vi "Drive Train.vi"(11 "Refnum in":refnum<k33>) -> ()   [LabVIEW 2014]
uses:
  TeleopCmd.ctl
  CmdFlag.ctl
  Drive Train Metrics.ctl
  <vilib>/Platform/TimedLoop/XDataNode/timing_clust.ctl
  <vilib>/Platform/TimedLoop/XDataNode/nitl_modes.ctl
  <vilib>/Platform/TimedLoop/XDataNode/wakeup.ctl
  <vilib>/platform/TimedLoop/XDataNode/XDataNode.xnode
  <vilib>/Platform/TimedLoop/XDataNode/XDNodeRunTimeDep.lvlib
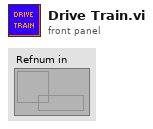
[diagram p1: front panel]
types:
  T1 = typedef "Drive Train Metrics.ctl" = cluster{"CmdFlag":T2, "Right Motor Power":dbl, "Left Motor Power":dbl, "Filtered Left Drive Rate":dbl, "Filtered Right Drive Rate":dbl, "Time of Last Metric":u32, "FIFO Timeout":i32, "Requested Left Velocity":dbl, "Requested Right Velocity":dbl, "throttle":dbl, "turn":dbl, "MaxDrivePwr":dbl, "Strafe":dbl, "Override":bool, "Time Of Last Turn":dbl, "Front_Strafe_Power":dbl, "Back_Strafe_Power":dbl, "MaxStrafePwr":dbl, "PrevMotorLevel":u8}
  T2 = typedef "CmdFlag.ctl" = enum16{"noop", "logflag", "suspend", "resume"}
  T3 = typedef "XDNodeRunTimeDep.lvlib/timing_clust.ctl" = cluster{"Expected End [f-1]":u64, "Actual End [f-1]":u64, "Finished Late? [f-1]":bool, "Expected End [i-1]":u64, "Actual End [i-1]":u64, "Finished Late? [i-1]":bool, "Expected Start [i]":u64, "Actual Start [i]":u64, "Expected Start [f]":u64, "Actual Start [f]":u64, "Source Name":string, "Structure Name":string, "Period":i64, "Deadline":i64, "Offset":i64, "Start":i64, "Priority":i32, "Timeout":i32, "Mode":T4, "Wakeup Reason":T5, "Error":errorcluster, "Source Type":string, "Secondary Source Type":string, "Global End Time":u64, "Global Start Time":u64, "Frame Duration":u64, "Iteration Duration":u64, "Assigned CPU":i32, "I/O Scan Engine Mode":u32}
  T4 = typedef "XDNodeRunTimeDep.lvlib/nitl_modes.ctl" = enum32{"No Change", "Process missed periods, maintain original phase", "Discard missed periods, maintain original phase", "Process missed periods, ignore original phase", "Discard missed periods, ignore original phase"}
  T5 = typedef "XDNodeRunTimeDep.lvlib/wakeup.ctl" = enum32{"Normal", "Aborted", "Asynchronous wakeup", "Timing source error", "Timed loop error", "Timeout"}
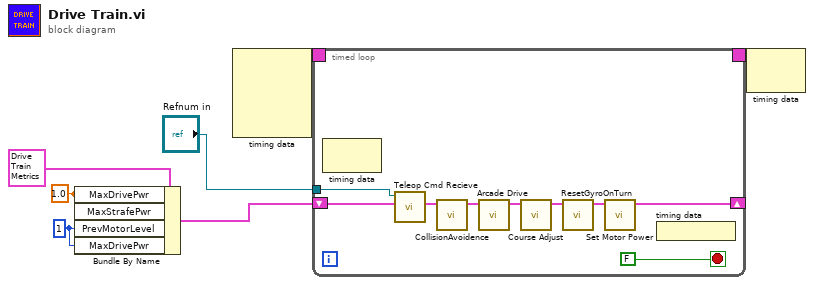
[diagram p0: block diagram]
diagram:
  w1 = u8 1 ("PrevMotorLevel")
  w2 = 1.0 ("MaxMotorPwr")
  n1 = Bundle By Name(cluster=T1 {"CmdFlag"=enum."noop", "Right Motor Power"=0.0, "Left Motor Power"=0.0, "Filtered Left Drive Rate"=0.0, "Filtered Right Drive Rate"=0.0, "Time of Last Metric"=0, "FIFO Timeout"=0, "Requested Left Velocity"=0.0, "Requested Right Velocity"=0.0, "throttle"=0.0, "turn"=0.0, "MaxDrivePwr"=0.0, "Strafe"=0.0, "Override"=FALSE, "Time Of Last Turn"=0.0, "Front_Strafe_Power"=0.0, "Back_Strafe_Power"=0.0, "MaxStrafePwr"=0.0, "PrevMotorLevel"=0} ("Cluster"), "MaxDrivePwr"=w2, "MaxStrafePwr"=w2, "PrevMotorLevel"=w1, "MaxDrivePwr"=w1) -> (w3:T1)
  n2 = node-c288() -> (w7:T3)  [unwired: 4 in]
  n3 = timed-loop {
    timing: w7 -> [_]
    timing-out: [_] -> w6
    tunnel: "Refnum in" -> [w11]
    shift-right: [w12] -> _
    shift-left: w3 -> [w10]
    stop <- FALSE stop-if-true
    n4 = node-c288() -> ()  [unwired: 1 in, 1 out]
    n5 = call "Teleop Cmd Recieve.vi"("Metrics Input"=w10, "rt fifo"=w11) -> ("Updated Drive Metrics"=w9:T1)  [unwired: 8 in, 1 out]
    n6 = call "CollisionAvoidence.vi"("Cluster"=w9) -> ("output cluster"=w8:T1)  [unwired: 10 in]
    n7 = call "Arcade Drive.vi"("Drive Metrics In"=w8) -> ("Drive Metrics out"=w15:T1)  [unwired: 10 in]
    n8 = call "Course Adjust.vi"("Drive Metrics In"=w15) -> ("Drive Train Metrics Out"=w14:T1)  [unwired: 10 in]
    n9 = call "ResetGyroOnTurn.vi"("Drive Train Metrics in"=w14) -> ("Drive Train Metrics Out"=w13:T1)  [unwired: 9 in]
    n10 = call "Set Motor Power.vi"("Drive Train Metrics In"=w13) -> ("Drive Train Metrics Out"=w12:T1)  [unwired: 9 in]
    n11 = node-c288() -> ()  [unwired: 1 out]
  }
  n12 = node-c288(w6) -> ()  [unwired: 1 out]
